vi "单路通断器（STR[]).vi"(1 "默认值":string, 2 "直通？":bool[](array[boolean]), 3 "X_In":string[](array[string])) -> (0 "X_Out":string[](array[string]))   [LabVIEW 2012]
doc: "功能：\n\n返回一个枚举，表明输入数的范围，用于三段比较。\n\n\nCSXCS_366创建。"
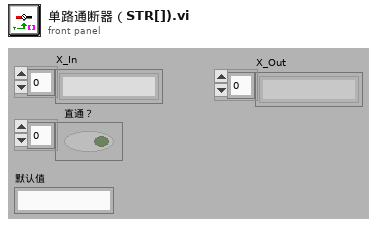
[diagram p1: front panel]
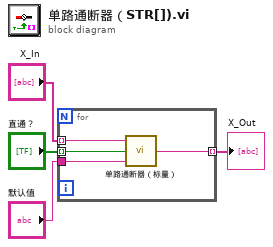
[diagram p0: block diagram]
diagram:
  n1 = for {
    tunnel: "X_In" -> [w8] mode=indexing
    tunnel: "直通？" -> [w7] mode=indexing
    tunnel: "默认值" -> [w6]
    tunnel: [w5] -> w1 mode=indexing
    n2 = call-poly "单路通断器（标量）.vi"("默认值"=w6, "直通？"=w7, "X_In"=w8) -> ("X_Out"=w5:string)
  }
  "X_Out" <- w1
